vi "SetSensorType.vi"(8 "error in (no error)":errorcluster) -> (0 "error out":errorcluster)   [LabVIEW 2015, in "ESLSCDLL.lvlib"]
uses:
  ESLSCDLL.lvlib
  Globals.vi
  ESLSCDLL.dll
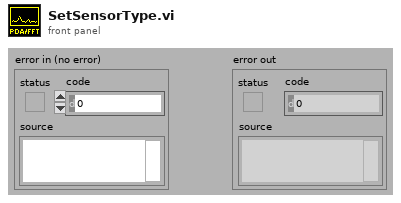
[diagram p1: front panel]
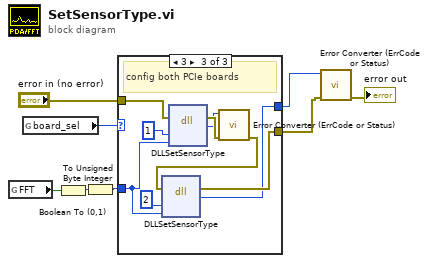
[diagram p0: block diagram]
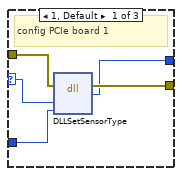
[diagram p2: hidden frame]
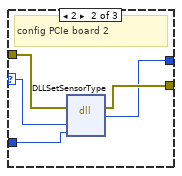
[diagram p3: hidden frame]
diagram:
  n1 = global read "Globals.vi" "FFT"() -> (w2:bool)
  n2 = global read "Globals.vi" "board_sel"() -> (w4:u32)
  n3 = Boolean To (0,1)(Boolean=w2) -> (0, 1=w3:i16)
  n4 = To Unsigned Byte Integer(number=w3) -> (unsigned 8bit integer=w1:u8)
  n5 = case shown="3" w4 {
    selector: w4 -> [w13 w18 _]
    tunnel: w1 -> [w12 w17 w25]
    tunnel: "error in (no error)" -> [w11 w16 w24]
    tunnel: [w10 w15 w20] -> w6
    tunnel: [w9 w14 w19] -> w5
    frame 1, Default {
      # "config PCIe board 1"
      n6 = dll-call lib="C:/Users/flori/Nextcloud/Dokumente/Stresing/Windows/lv64/board.vis/ESLSCDLL.dll" fn="DLLSetSensorType" ("lwlscdll.dll:DLLSetISPDA")(error in=w11, "drv"=w13, "sensor_type"=w12) -> (error out=w10:errorcluster, "es_status_codes"=w9:i32)  [unwired: 4 in, 1 out]
    }
    frame 2 {
      # "config PCIe board 2"
      n7 = dll-call lib="C:/Users/flori/Nextcloud/Dokumente/Stresing/Windows/lv64/board.vis/ESLSCDLL.dll" fn="DLLSetSensorType" ("lwlscdll.dll:DLLSetISPDA")(error in=w16, "drv"=w18, "sensor_type"=w17) -> (error out=w15:errorcluster, "es_status_codes"=w14:i32)  [unwired: 4 in, 1 out]
    }
    frame 3 {
      # "config both PCIe boards"
      n8 = dll-call lib="C:/Users/flori/Nextcloud/Dokumente/Stresing/Windows/lv64/board.vis/ESLSCDLL.dll" fn="DLLSetSensorType" ("lwlscdll.dll:DLLSetISPDA")(error in=w24, "drv"=u32 1, "sensor_type"=w25) -> (error out=w23:errorcluster, "es_status_codes"=w22:i32)  [unwired: 4 in, 1 out]
      n9 = call "Error Converter (ErrCode or Status).vi"("error in (no error)"=w23, "error code"=w22) -> ("error out"=w21:errorcluster)  [unwired: 9 in]
      n10 = dll-call lib="C:/Users/flori/Nextcloud/Dokumente/Stresing/Windows/lv64/board.vis/ESLSCDLL.dll" fn="DLLSetSensorType" ("lwlscdll.dll:DLLSetISPDA")(error in=w21, "drv"=u32 2, "sensor_type"=w25) -> (error out=w20:errorcluster, "es_status_codes"=w19:i32)  [unwired: 4 in, 1 out]
    }
  }
  n11 = call "Error Converter (ErrCode or Status).vi"("error in (no error)"=w6, "error code"=w5) -> ("error out"=→"error out":errorcluster)  [unwired: 9 in]
